vi "queue-3.vi"() -> ()   [LabVIEW 2010]
panel:
  out "Numeric":i32
  in  "stop":bool
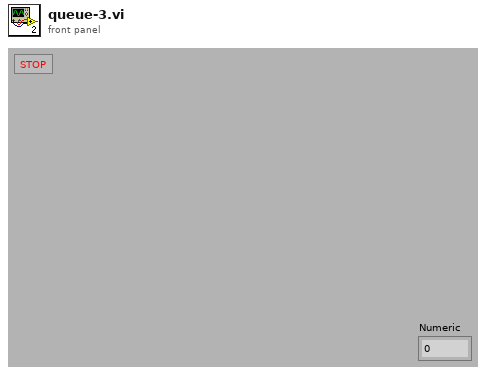
[diagram p1: front panel]
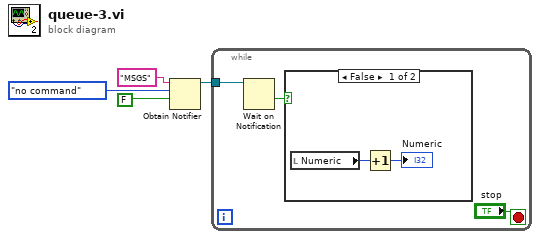
[diagram p0: block diagram]
diagram:
  n1 = Obtain Notifier(name (unnamed)="MSGS", notification data type=enum16{"no command", "refresh"}."no command", create if not found? (T)=FALSE) -> (notifier out=w2:refnum<notifier>)  [unwired: 1 in, 2 out]
  n2 = while {
    tunnel: w2 -> [w6]
    stop <- "stop" stop-if-true
    n3 = Wait on Notification(notifier=w6) -> (timed out?=w5:bool)  [unwired: 3 in, 3 out]
    n4 = case shown="False" w5 {
      frame False {
        n5 = local read "Numeric"() -> (w9:i32)
        n6 = Increment(x=w9) -> (x+1=→"Numeric":i32)
      }
      frame True {
      }
    }
  }
